vi "fo.vi"(1 "q_input":dbl[](array[numeric]), 2 "object cluster":T1) -> (0 "fo":dbl)   [LabVIEW 2019]
panel:
  # "input : object cluster\n             q_input"
  # "output : fo, double"
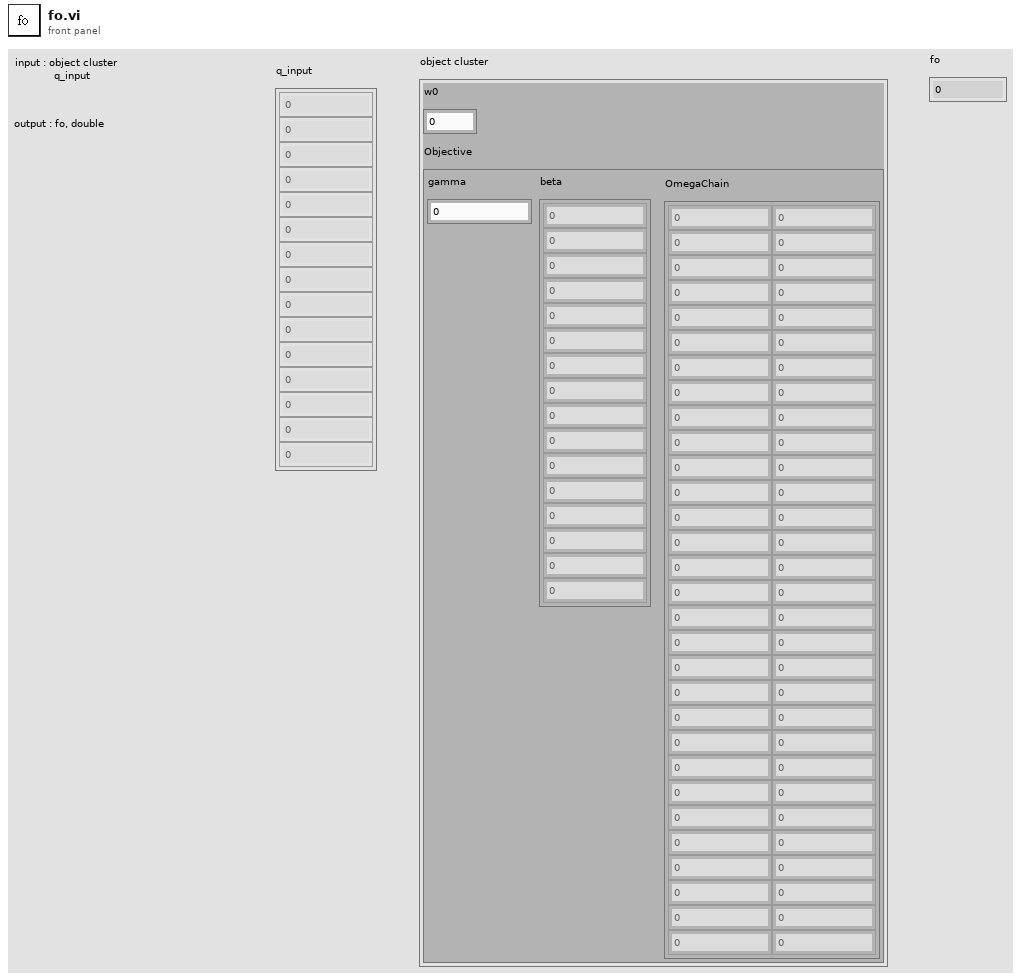
[diagram p1: front panel]
types:
  T1 = cluster{"w0":dbl, "Objective":cluster{"beta":dbl[], "gamma":dbl, "OmegaChain":dbl[][]}}
  T2 = cluster{"beta":dbl[], "gamma":dbl, "OmegaChain":dbl[][]}
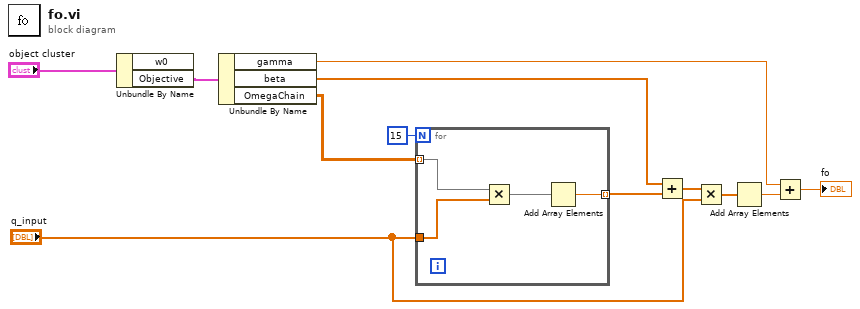
[diagram p0: block diagram]
diagram:
  n1 = Unbundle By Name("object cluster") -> ("Objective"=w10:T2)  [unwired: 1 out]
  n2 = Unbundle By Name(w10) -> ("gamma"=w2:dbl, "beta"=w3:dbl[], "OmegaChain"=w8:dbl[][])
  n3 = for {
    N: 15 -> [_]
    tunnel: "q_input" -> [w13]
    tunnel: [w15] -> w7 mode=indexing
    tunnel: w8 -> [w14] mode=indexing
    n4 = Multiply(x=w14, y=w13) -> (x*y=w16:dbl[])
    n5 = Add Array Elements(numeric array=w16) -> (sum=w15:dbl)
  }
  n6 = Add(x=w3, y=w7) -> (x+y=w6:dbl[])
  n7 = Multiply(x=w6, y="q_input") -> (x*y=w5:dbl[])
  n8 = Add Array Elements(numeric array=w5) -> (sum=w4:dbl)
  n9 = Add(x=w2, y=w4) -> (x+y=→"fo":dbl)
